vi "Parameters_file_v01.vi"(4 "Additional text":string, 5 "actual sample rate array":dbl[](array[numeric]), 6 "actualSamples array":i32[](array[numeric]), 7 "Files name array":string[](array[string]), 8 "File location":path, 9 "Record":bool) -> (0 "Full text":string)   [LabVIEW 2013]
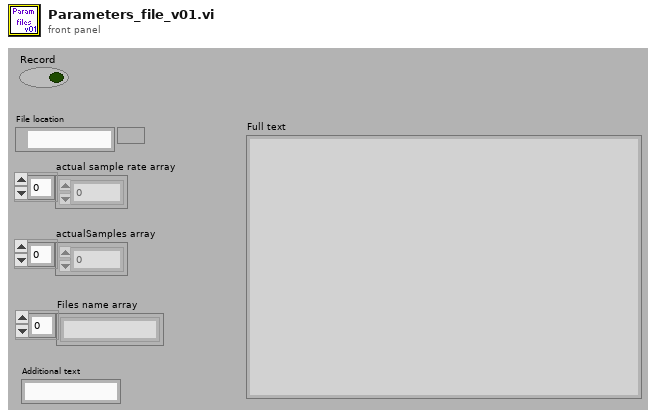
[diagram p1: front panel]
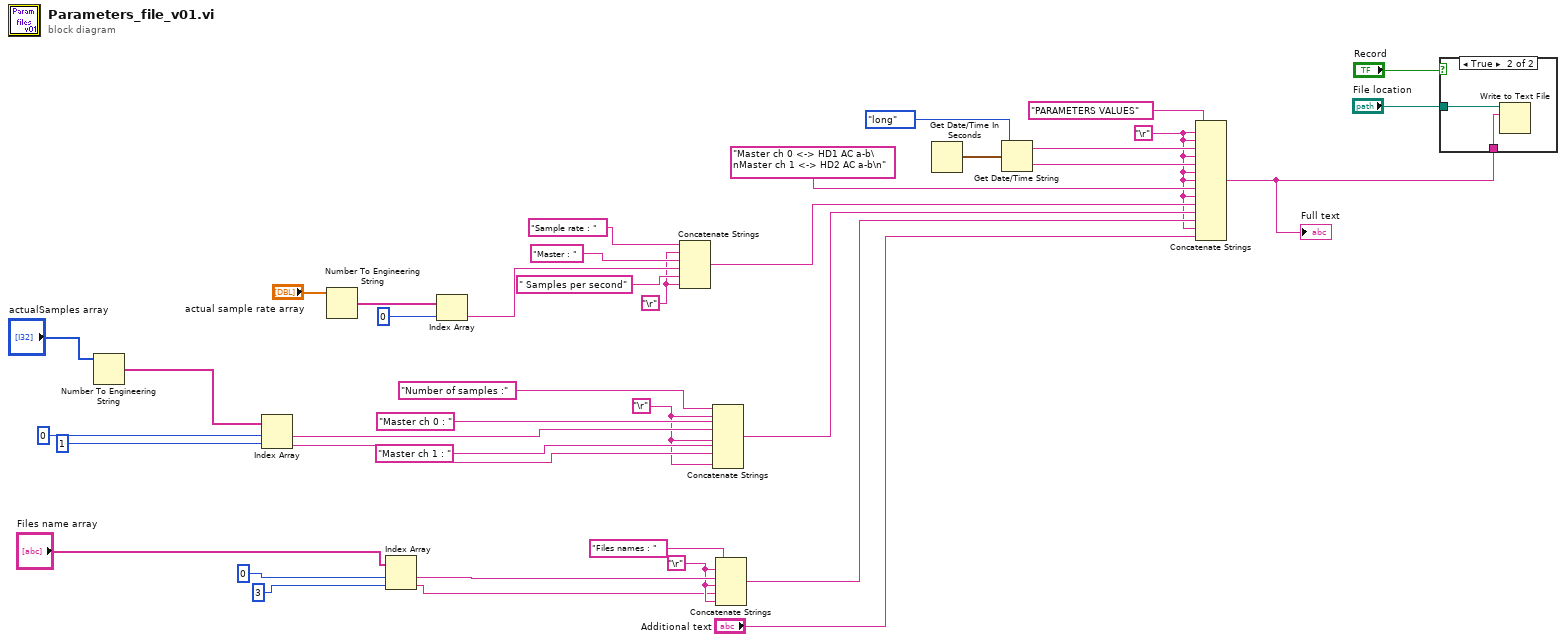
[diagram p0: block diagram]
diagram:
  w11 = "\r"
  w9 = "\r"
  w4 = "\r"
  w1 = "\r"
  n1 = Number To Engineering String(4:"actualSamples array") -> (0:w29:string[])  [unwired: 3 out]
  n2 = Index Array(array=w29, index #1=0 ("index"), index #2=1 ("index")) -> (element #1=w23:string, element #2=w21:string)
  n3 = Number To Engineering String(4:"actual sample rate array") -> (0:w16:string[])  [unwired: 3 out]
  n4 = Index Array(array="Files name array", index #1=0 ("index"), index #2=3 ("index")) -> (element #1=w5:string, element #2=w3:string)
  n5 = Index Array(array=w16, index=0) -> (element=w13:string)
  n6 = Concatenate Strings("Sample rate : " ("string"), w11, "Master : " ("string"), w13, " Samples per second" ("string"), w11) -> (w20:string)
  n7 = Concatenate Strings("Number of samples :" ("string"), w9, "Master ch 0 : " ("string"), w23, w9, "Master ch 1 : " ("string"), w21, w9) -> (w19:string)
  n8 = Concatenate Strings("Files names : " ("string"), w4, w5, w4, w3, w4) -> (w18:string)
  n9 = Get Date/Time In Seconds() -> (seconds since 1Jan1904=w36:timestamp)
  n10 = Get Date/Time String(date format (0)=enum16{"short", "long", "abbreviated"}."long", seconds (now)=w36) -> (date string=w33:string, time string=w35:string)  [unwired: 1 out]
  n11 = Concatenate Strings("PARAMETERS VALUES" ("string"), w1, w1, w33, w1, w35, w1, w1, "Master ch 0 <-> HD1 AC a-b\nMaster ch 1 <-> HD2 AC a-b\n", w1, w20, w19, w18, w1, "Additional text") -> (w37:string)
  "Full text" <- w37
  n12 = case shown="True" "Record" {
    tunnel: "File location" -> [_ w41]
    tunnel: w37 -> [_ w40]
    frame False {
    }
    frame True {
      n13 = Write to Text File(file (use dialog)=w41, text=w40) -> ()  [unwired: 1 in, 4 out]
    }
  }
